vi "Convert with Linear Calibration (1D, DBL array).vi"(10 "Linear Calibration 1D":T1, 11 "A":dbl[](array[numeric])) -> (3 "A*":dbl[](array[numeric]))   [LabVIEW 2011, in "COSYLib.lvlib"]
doc: "Calculates Y=AX+B, with A and B taken from a <B>Linear Calibration</B> cluster."
uses:
  COSYLib.lvlib
  Linear Calibration 1D.ctl
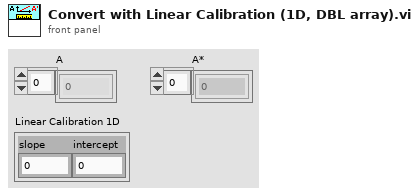
[diagram p1: front panel]
types:
  T1 = typedef "COSYLib.lvlib/Linear Calibration 1D.ctl" = cluster{"slope":dbl, "intercept":dbl}
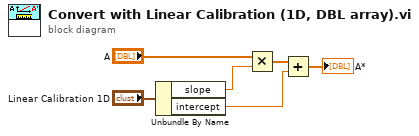
[diagram p0: block diagram]
diagram:
  n1 = Unbundle By Name("Linear Calibration 1D") -> ("slope"=w5:dbl, "intercept"=w3:dbl)
  n2 = Multiply(x="A", y=w5) -> (x*y=w4:dbl[])
  n3 = Add(x=w4, y=w3) -> (x+y=→"A*":dbl[])
